vi "stderr.vi"() -> (0 "stderr":path)   [LabVIEW 2014]
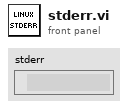
[diagram p1: front panel]
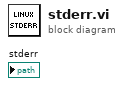
[diagram p0: block diagram]
diagram:
